vi "Fault Code.vi"(8 "error in (no error)":errorcluster, 11 "Fault Code":i32) -> (0 "error out":errorcluster, 2 "Fault Cluster":T1)   [LabVIEW 2016]
uses:
  sniper current tests/Fault Cluster.ctl
panel:
  in  "Mask Unused?":bool=TRUE
  out "Fault Code 2":i32
  out "Unused status are 0s":i16 format="0b%16b"
  in  "Unused status are 1s":i16=-28576 format="0b%16b"
  out "size(s) 2":i32
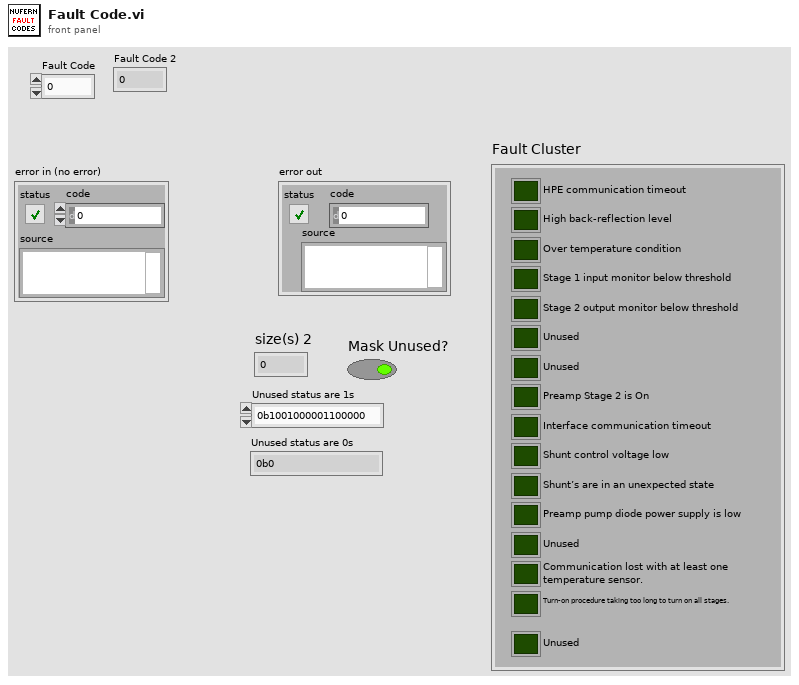
[diagram p1: front panel]
types:
  T1 = typedef "Fault Cluster.ctl" = cluster{"HPE communication timeout":bool, "High back-reflection level":bool, "Over temperature condition":bool, "Stage 1 input monitor below threshold":bool, "Stage 2 output monitor below threshold":bool, "Unused":bool, "Unused":bool, "Preamp Stage 2 is On":bool, "Interface communication timeout":bool, "Shunt control voltage low":bool, "Shunt’s are in an unexpected state":bool, "Preamp pump diode power supply is low":bool, "Unused":bool, "Communication lost with at least one\ntemperature sensor.":bool, "Turn-on procedure taking too long to turn on all stages.":bool, "Unused":bool}
  T2 = cluster{"[0]":bool, "[1]":bool, "[2]":bool, "[3]":bool, "[4]":bool, "[5]":bool, "[6]":bool, "[7]":bool, "[8]":bool, "[9]":bool, "[10]":bool, "[11]":bool, "[12]":bool, "[13]":bool, "[14]":bool, "[15]":bool}
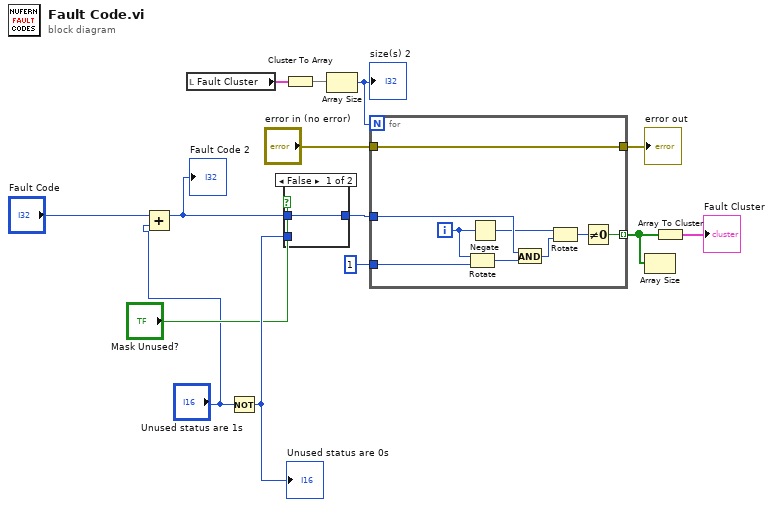
[diagram p0: block diagram]
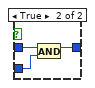
[diagram p2: hidden frame]
diagram:
  n1 = Add(x="Fault Code", y="Unused status are 1s") -> (x+y=w3:i32)
  "Fault Code 2" <- w3
  n2 = local read "Fault Cluster"() -> (w6:T1)
  n3 = Not(x="Unused status are 1s") -> (.not. x?=w4:i16)
  "Unused status are 0s" <- w4
  n4 = case shown="False" "Mask Unused?" {
    tunnel: [w15 w18] -> w5
    tunnel: w4 -> [_ w17]
    tunnel: w3 -> [w15 w16]
    frame False {
    }
    frame True {
      n5 = And(x=w16, y=w17) -> (x .and. y?=w18:i32)
    }
  }
  n6 = Cluster To Array(cluster=w6) -> (array=w13:bool[])
  n7 = Array Size(array=w13) -> (size(s)=w12:i32)
  "size(s) 2" <- w12
  n8 = for {
    N: w12 -> [_]
    tunnel: "error in (no error)" -> [w27]
    tunnel: [w27] -> w8
    tunnel: w5 -> [w26]
    tunnel: 1 -> [w25]
    tunnel: [w19] -> w11 mode=indexing
    i -> [w22]
    n9 = Rotate(1:w25, 2:w22) -> (0:w24:i32)
    n10 = Negate(x=w22) -> (-x=w21:i32)
    n11 = And(x=w26, y=w24) -> (x .and. y?=w23:i32)
    n12 = Rotate(1:w23, 2:w21) -> (0:w20:i32)
    n13 = Not Equal To 0?(x=w20) -> (x != 0?=w19:bool)
  }
  "error out" <- w8
  n14 = Array Size(array=w11) -> ()  [unwired: 1 out]
  n15 = Array To Cluster(array=w11) -> (cluster=→"Fault Cluster":T2)
